vi "LH6Checksum_inycom.vi"(8 "error in":errorcluster, 11 "Data in":string[](array[string])) -> (0 "error out":errorcluster, 3 "Data out":string[](array[string]))   [LabVIEW 2015]
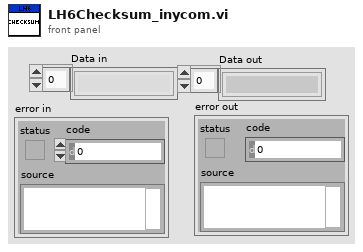
[diagram p1: front panel]
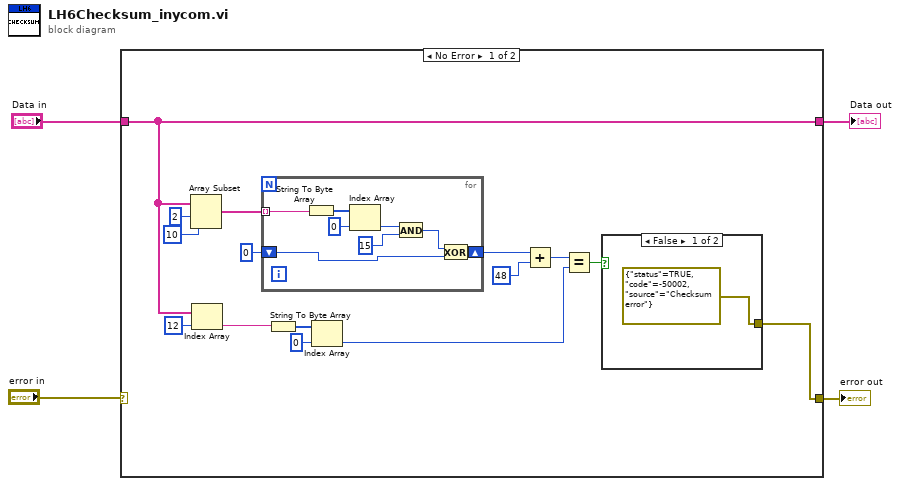
[diagram p0: block diagram]
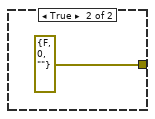
[diagram p2: hidden frame]
diagram:
  n1 = case shown="No Error" "error in" {
    selector: "error in" -> [_ w31]
    tunnel: "Data in" -> [w7 w30]
    tunnel: [w5 w31] -> w2
    tunnel: [w7 w30] -> w1
    frame No Error {
      n2 = Array Subset(array=w7, index=2, length=10) -> (w11:string[])
      n3 = Index Array(array=w7, index=12) -> (element=w17:string)
      n4 = for {
        tunnel: w11 -> [w29] mode=indexing
        shift-right: [w23] -> w12
        shift-left: u8 0 -> [w22]
        n5 = String To Byte Array(string=w29) -> (unsigned byte array=w28:u8[])
        n6 = Index Array(array=w28, index=0) -> (element=w26:u8)
        n7 = And(x=w26, y=u8 15) -> (x .and. y?=w24:u8)
        n8 = Exclusive Or(1:w22, 2:w24) -> (0:w23:u8)
      }
      n9 = String To Byte Array(string=w17) -> (unsigned byte array=w15:u8[])
      n10 = Index Array(array=w15, index=0) -> (element=w19:u8)
      n11 = Add(x=w12, y=u8 48) -> (x+y=w18:u8)
      n12 = Equal?(x=w18, y=w19) -> (x = y?=w6:bool)
      n13 = case shown="False" w6 {
        tunnel: [errorcluster {"status"=TRUE, "code"=-50002, "source"="Checksum error"} ("error IO") errorcluster {"status"=FALSE, "code"=0, "source"=""} ("error IO")] -> w5
        frame False {
        }
        frame True {
        }
      }
    }
    frame Error {
    }
  }
  "error out" <- w2
  "Data out" <- w1
